vi "Initialize Waveforms V4.vi"(0 "Image Acquisition Parameters":T2={"Scan Type"=enum."Sample Scanning", "Scan Mode"=enum."XY", "Fast Axis Frequency (Hz)"=100.0, "Image Format"=128, "Line Accumulations"=1, "Frames Per Capture"=1, "Frames Accumulations"=1, "Image Dimension (um)"=[], "Number of Z Steps"=1, "Z Steps Size (um)"=1.0, "Pixel Size (nm)"=[], "Customized Image Format"=[]} {"Z Steps Size (um)" min=0.0; "Number of Z Steps" min=1; "Frames Accumulations" min=1; "Frames Per Capture" min=1; "Line Accumulations" min=1; "Image Format" items=["64 x 64"=64, "128 x 128"=128, "256 x 256"=256, "512 x 512"=512, "1024 x 1024"=1024, "2048 x 2048"=2048, "Customized..."=0]}) -> (4 "Waveform Data to FPGA":T1)   [LabVIEW 2014]
uses:
  Type Defs/Image Acquisition Parameters.ctl
  Waveform Data.ctl
panel:
  in  "Slow Axis 2 Delay (Galvo - Not YZ)":i32=2
  in  "Number Data of Points":i32=5000
  # "Length"
  # "Height"
  # "XY"
  # "Z"
  # "Length"
  # "Height"
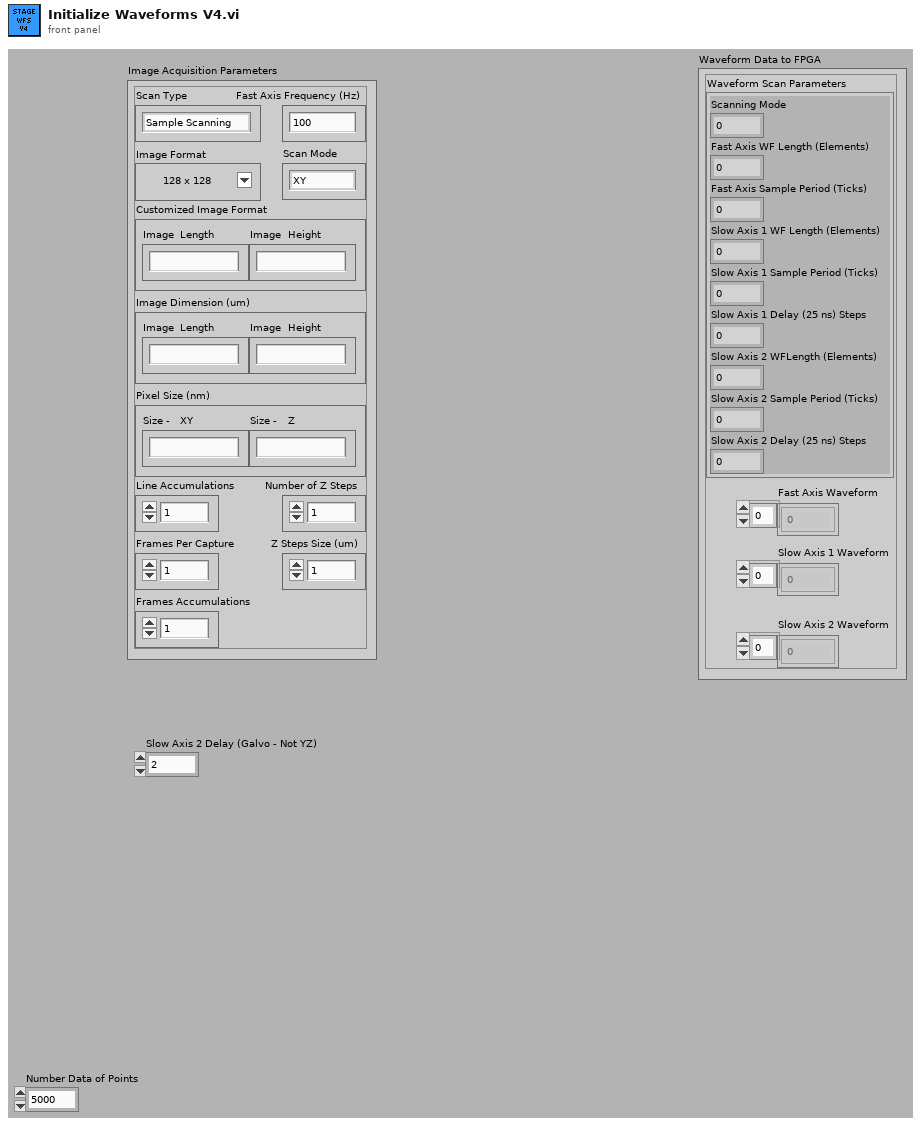
[diagram p1: front panel]
types:
  T1 = typedef "Waveform Data.ctl" = cluster{"Waveform Scan Parameters":cluster{"Scanning Mode":u8, "Fast Axis WF Length (Elements)":i32, "Fast Axis Sample Period (Ticks)":u32, "Slow Axis 1 WF Length (Elements)":i32, "Slow Axis 1 Sample Period (Ticks)":u32, "Slow Axis 1 Delay (25 ns) Steps":i32, "Slow Axis 2 WFLength (Elements)":i32, "Slow Axis 2 Sample Period (Ticks)":u32, "Slow Axis 2 Delay (25 ns) Steps":i32}, "Fast Axis Waveform":dbl[], "Slow Axis 1 Waveform":dbl[], "Slow Axis 2 Waveform":dbl[]}
  T2 = typedef "Image Acquisition Parameters.ctl" = cluster{"Scan Type":enum16{"Sample Scanning", "Beam Scanning"}, "Scan Mode":enum16{"XY", "XZ", "YZ", "XYZ"}, "Fast Axis Frequency (Hz)":dbl, "Image Format":u16, "Line Accumulations":u16, "Frames Per Capture":u16, "Frames Accumulations":u16, "Image Dimension (um)":dbl[], "Number of Z Steps":u8, "Z Steps Size (um)":dbl, "Pixel Size (nm)":dbl[], "Customized Image Format":dbl[]}
  T3 = cluster{"Scanning Mode":u8, "Fast Axis WF Length (Elements)":i32, "Fast Axis Sample Period (Ticks)":u32, "Slow Axis 1 WF Length (Elements)":i32, "Slow Axis 1 Sample Period (Ticks)":u32, "Slow Axis 1 Delay (25 ns) Steps":i32, "Slow Axis 2 WFLength (Elements)":i32, "Slow Axis 2 Sample Period (Ticks)":u32, "Slow Axis 2 Delay (25 ns) Steps":i32}
  T4 = typedef "Scan Parameters.ctl" = cluster{"Fast_Ax_Amp_V":dbl, "Fast_Ax_Off_V":dbl, "Slow_Ax_Amp_V":dbl, "Slow_Ax_Off_V ":dbl, "Slow_Ax_Max_V_VperS":dbl, "Slow_Ax1_Del25ns":i32, "Slow_Ax2_Del25ns":i32, "Stage_X_Off_V":dbl, "Stage_Y_Off_V":dbl, "Stage_Z_Off_V":dbl, "Galvo1_Off_V":dbl, "Galvo2_Off_V":dbl, "Last_Scan_Mode":enum16{"XY", "XZ", "YZ", "XYZ"}, "Current_Scan_Mode":enum16{"XY", "XZ", "YZ", "XYZ"}, "Fly_Back_Lines":u16, "Linear_Ramp_End":u32, "Z_Step_I16":i16, "Z_Start_I16":i16, "Laser_States _U32":u32, "590_Voltage_I16":i16, "775_AOM_Volt_I16":i16, "Blanking OFF":bool, "Unused_Axis_I16":i16}
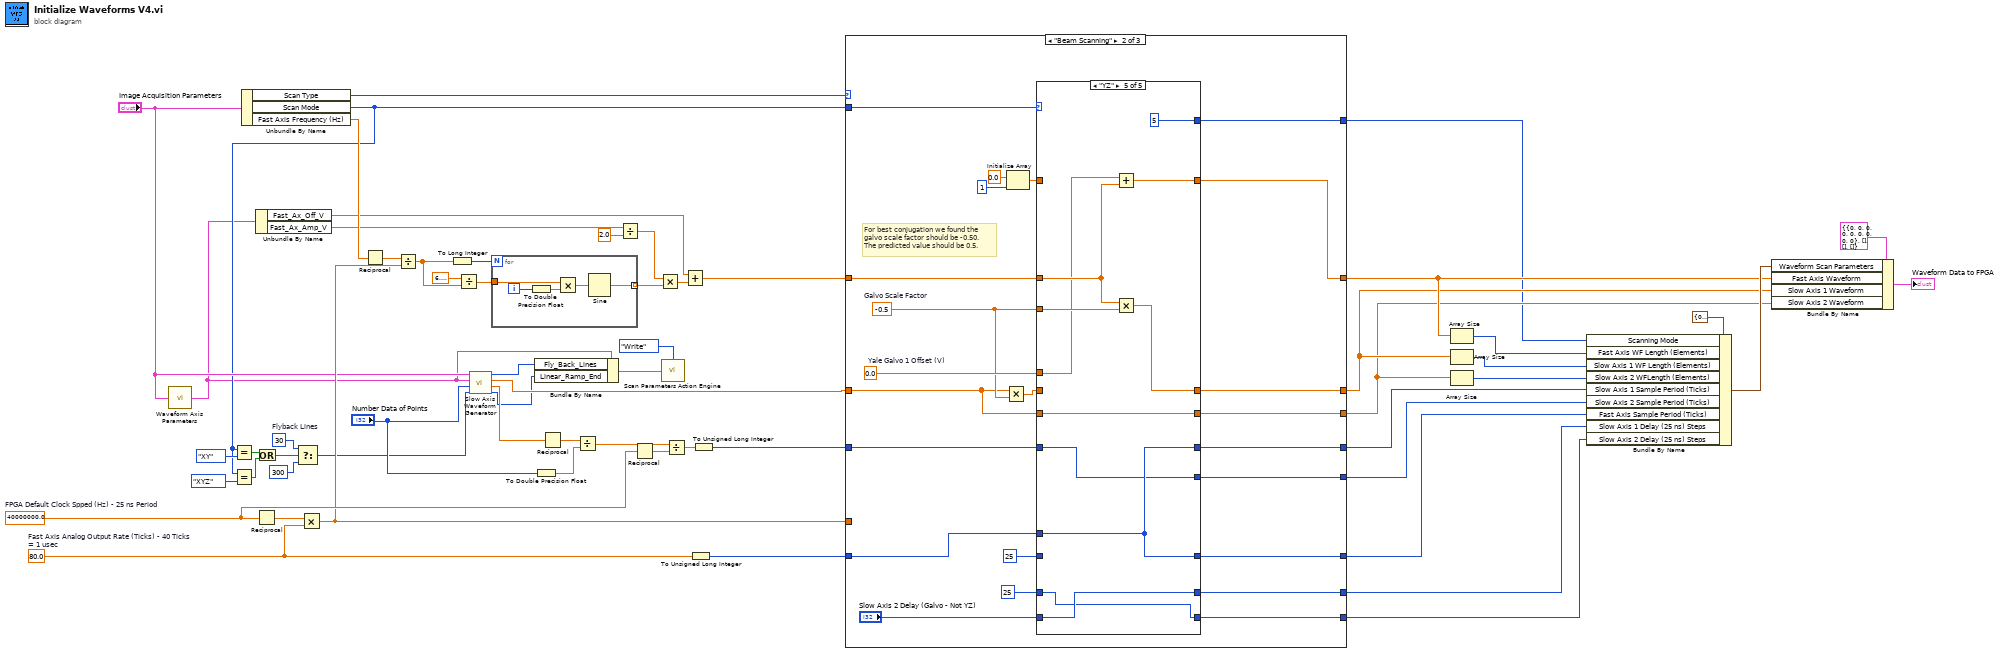
[diagram p0: block diagram]
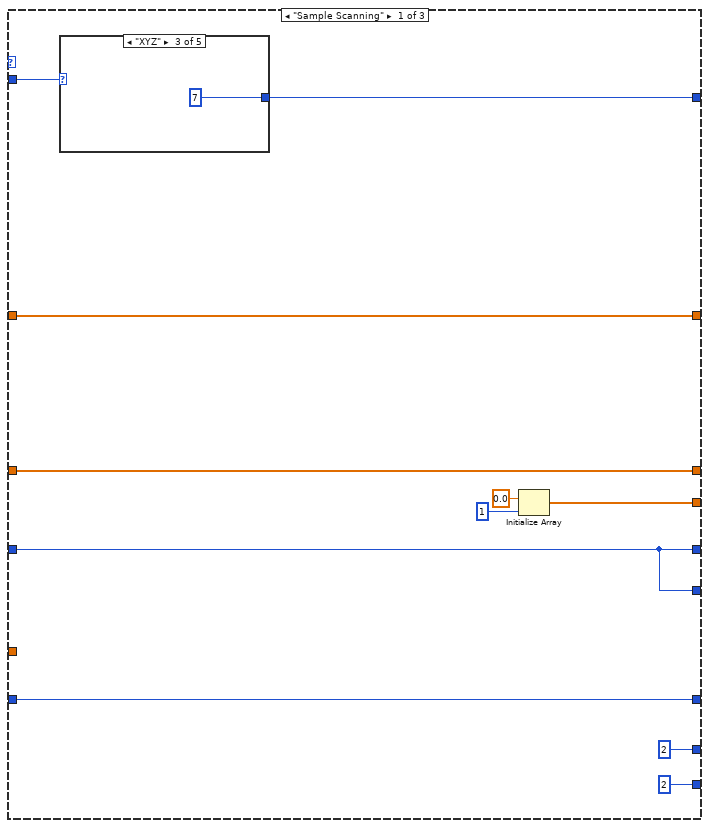
[diagram p2: hidden frame]
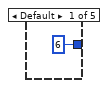
[diagram p3: hidden frame]
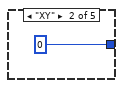
[diagram p4: hidden frame]
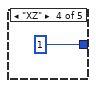
[diagram p5: hidden frame]
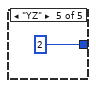
[diagram p6: hidden frame]
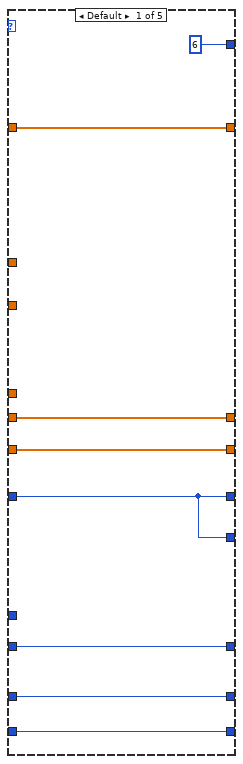
[diagram p7: hidden frame]
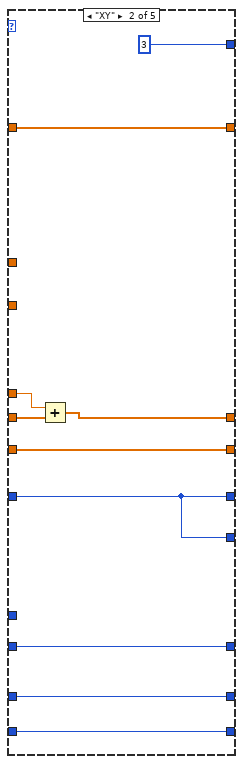
[diagram p8: hidden frame]
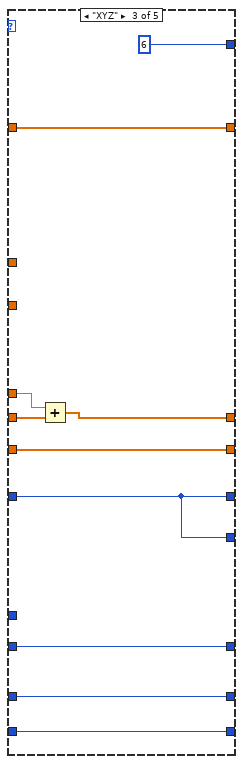
[diagram p9: hidden frame]
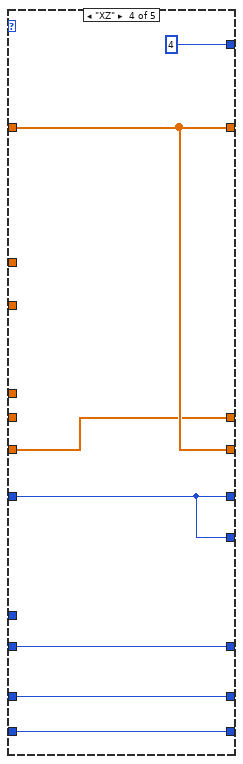
[diagram p10: hidden frame]
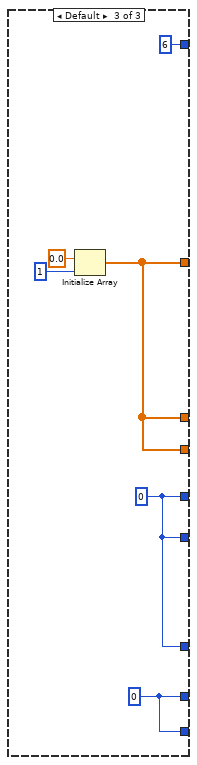
[diagram p11: hidden frame]
diagram:
  w10 = u16 30  # Flyback Lines
  w36 = 80.0  # Fast Axis Analog Output Rate (Ticks) - 40 Ticks = 1 usec
  w46 = 40000000.0  # FPGA Default Clock Spped (Hz) - 25 ns Period
  n1 = call "Waveform Axis Parameters.vi"("Image Acquisition Parameters"="Image Acquisition Parameters") -> ("Scan Parameters"=w1:T4)  [unwired: 14 in]
  n2 = Unbundle By Name("Image Acquisition Parameters") -> ("Scan Type"=w51:enum16{"Sample Scanning", "Beam Scanning"}, "Scan Mode"=w2:enum16{"XY", "XZ", "YZ", "XYZ"}, "Fast Axis Frequency (Hz)"=w21:dbl)
  n3 = Equal?(x=w2, y=enum16{"XY", "XZ", "YZ", "XYZ"}."XY") -> (x = y?=w6:bool)
  n4 = Equal?(x=w2, y=enum16{"XY", "XZ", "YZ", "XYZ"}."XYZ") -> (x = y?=w5:bool)
  n5 = Unbundle By Name(w1) -> ("Fast_Ax_Off_V"=w18:dbl, "Fast_Ax_Amp_V"=w19:dbl)
  n6 = Reciprocal(x=w46) -> (1/x=w50:dbl)
  n7 = Or(x=w6, y=w5) -> (x .or. y?=w4:bool)
  n8 = Select(t=w10, s=w4, f=u16 300) -> (s? t:f=w3:u16)
  n9 = Multiply(x=w50, y=w36) -> (x*y=w16:dbl)
  n10 = Reciprocal(x=w21) -> (1/x=w26:dbl)
  n11 = Divide(x=w26, y=w16) -> (x/y=w24:dbl)
  n12 = To Long Integer(number=w24) -> (32bit integer=w25:i32)
  n13 = Divide(x=6.283185307179586, y=w24) -> (x/y=w29:dbl)
  n14 = call "Slow Axis Waveform Generator.vi"("Flyback Lines"=w3, "Number Data of Points"="Number Data of Points", "Scan Parameters"=w1, "Image Acquisition Parameters"="Image Acquisition Parameters") -> ("Linear Ramp End"=w12:u32, "Slow Axis Frequency"=w48:dbl, "Slow Axis Waveform"=w49:dbl[], "Flyback Lines"=w15:u16)
  n15 = for {
    N: w25 -> [_]
    tunnel: w29 -> [w64]
    tunnel: [w61] -> w28 mode=indexing
    i -> [w60]
    n16 = To Double Precision Float(number=w60) -> (double precision float=w63:dbl)
    n17 = Multiply(x=w64, y=w63) -> (x*y=w62:dbl)
    n18 = Sine(x=w62) -> (sin(x)=w61:dbl)
  }
  n19 = Bundle By Name(cluster=w1, "Fly_Back_Lines"=w15, "Linear_Ramp_End"=w12) -> (w13:T4)
  n20 = To Double Precision Float(number="Number Data of Points") -> (double precision float=w55:dbl)
  n21 = Reciprocal(x=w48) -> (1/x=w56:dbl)
  n22 = Divide(x=w56, y=w55) -> (x/y=w54:dbl)
  n23 = Divide(x=w19, y=2.0) -> (x/y=w22:dbl)
  n24 = Reciprocal(x=w46) -> (1/x=w53:dbl)
  n25 = Multiply(x=w22, y=w28) -> (x*y=w27:dbl[])
  n26 = call "Scan Parameters Action Engine.vi"("Action"=enum16{"Read", "Write"}."Write", "Scan Parameters IN"=w13) -> ()  [unwired: 13 in, 1 out]
  n27 = Divide(x=w54, y=w53) -> (x/y=w52:dbl)
  n28 = Add(x=w18, y=w27) -> (x+y=w20:dbl[])
  n29 = To Unsigned Long Integer(number=w36) -> (unsigned 32bit integer=w35:u32)
  n30 = To Unsigned Long Integer(number=w52) -> (unsigned 32bit integer=w45:u32)
  n31 = case shown="\"Beam Scanning\"" w51 {
    tunnel: w2 -> [w75 w103 _]
    tunnel: w16 -> [_ _ _]
    tunnel: [w65 w101 w152] -> w43
    tunnel: w49 -> [w74 w81 _]
    tunnel: [w74 w97 w152] -> w42
    tunnel: [w71 w96 w152] -> w41
    tunnel: w45 -> [w68 w87 _]
    tunnel: [w70 w102 u8 6 ("Scanning Mode")] -> w37
    tunnel: w35 -> [w69 w84 _]
    tunnel: [w69 w93 w151] -> w34
    tunnel: [w68 w86 w151] -> w33
    tunnel: [w68 w85 w151] -> w32
    tunnel: [2 ("Slow Axis 2 Delay (25 ns) Steps") w92 w150] -> w31
    tunnel: [2 ("Slow Axis 2 Delay (25 ns) Steps") w90 w150] -> w17
    tunnel: w20 -> [w65 w94 _]
    frame "Sample Scanning" {
      n32 = case shown="\"XYZ\"" w75 {
        tunnel: [u8 6 ("Scanning Mode") u8 0 ("Scanning Mode") u8 7 ("Scanning Mode") u8 1 ("Scanning Mode") u8 2 ("Scanning Mode")] -> w70
        frame Default {
        }
        frame "XY" {
        }
        frame "XYZ" {
        }
        frame "XZ" {
        }
        frame "YZ" {
        }
      }
      n33 = Initialize Array(0.0 ("element"), 1 ("dimension size")) -> (w71:dbl[])
    }
    frame "Beam Scanning" {
      w82 = -0.5  # Galvo Scale Factor
      w95 = 0.0  # Yale Galvo 1 Offset (V)
      # "For best conjugation we found the\ngalvo scale factor should be -0.50.\nThe predicted value should be 0.5."
      n34 = Multiply(x=w81, y=w82) -> (x*y=w83:dbl[])
      n35 = Initialize Array(0.0 ("element"), 1 ("dimension size")) -> (w98:dbl[])
      n36 = case shown="\"YZ\"" w103 {
        tunnel: [u8 6 ("Scanning Mode") u8 3 ("Scanning Mode") u8 6 ("Scanning Mode") u8 4 ("Scanning Mode") u8 5 ("Scanning Mode")] -> w102
        tunnel: [w110 w120 w130 w137 w144] -> w101
        tunnel: w98 -> [w110 w120 w130 w137 _]
        tunnel: [w109 w117 w127 w132 w148] -> w97
        tunnel: w83 -> [w109 w118 w128 _ _]
        tunnel: w81 -> [w108 w119 w129 w132 w139]
        tunnel: [w108 w119 w129 w137 w139] -> w96
        tunnel: w95 -> [_ w116 w126 _ w145]
        tunnel: w94 -> [_ _ _ _ w146]
        tunnel: w82 -> [_ _ _ _ w147]
        tunnel: [w107 w115 w125 w135 w142] -> w93
        tunnel: u32 25 -> [w107 w115 w125 w135 _]
        tunnel: [w105 w114 w124 w133 w140] -> w92
        tunnel: "Slow Axis 2 Delay (Galvo - Not YZ)" -> [w105 w114 w124 w133 w143]
        tunnel: [w106 w113 w123 w134 w143] -> w90
        tunnel: 25 ("Slow Axis 1 Delay (25 ns) Steps") -> [w106 w113 w123 w134 w140]
        tunnel: [w104 w112 w122 w136 w142] -> w86
        tunnel: w87 -> [w104 w112 w122 w136 w141]
        tunnel: [w104 w112 w122 w136 w141] -> w85
        tunnel: w84 -> [_ _ _ _ w142]
        frame Default {
        }
        frame "XY" {
          n37 = Add(x=w116, y=w118) -> (x+y=w117:dbl[])
        }
        frame "XYZ" {
          n38 = Add(x=w126, y=w128) -> (x+y=w127:dbl[])
        }
        frame "XZ" {
        }
        frame "YZ" {
          n39 = Add(x=w145, y=w146) -> (x+y=w144:dbl[])
          n40 = Multiply(x=w146, y=w147) -> (x*y=w148:dbl[])
        }
      }
    }
    frame Default {
      w150 = 0 ("Slow Axis 2 Delay (25 ns) Steps")
      w151 = u32 0
      n41 = Initialize Array(0.0 ("element"), 1 ("dimension size")) -> (w152:dbl[])
    }
  }
  n42 = Array Size(array=w43) -> (size(s)=w40:i32)
  n43 = Array Size(array=w42) -> (size(s)=w39:i32)
  n44 = Array Size(array=w41) -> (size(s)=w38:i32)
  n45 = Bundle By Name(cluster=T3 {"Scanning Mode"=0, "Fast Axis WF Length (Elements)"=0, "Fast Axis Sample Period (Ticks)"=0, "Slow Axis 1 WF Length (Elements)"=0, "Slow Axis 1 Sample Period (Ticks)"=0, "Slow Axis 1 Delay (25 ns) Steps"=0, "Slow Axis 2 WFLength (Elements)"=0, "Slow Axis 2 Sample Period (Ticks)"=0, "Slow Axis 2 Delay (25 ns) Steps"=0} ("Waveform Scan Parameters"), "Scanning Mode"=w37, "Fast Axis WF Length (Elements)"=w40, "Slow Axis 1 WF Length (Elements)"=w39, "Slow Axis 2 WFLength (Elements)"=w38, "Slow Axis 1 Sample Period (Ticks)"=w33, "Slow Axis 2 Sample Period (Ticks)"=w32, "Fast Axis Sample Period (Ticks)"=w34, "Slow Axis 1 Delay (25 ns) Steps"=w17, "Slow Axis 2 Delay (25 ns) Steps"=w31) -> (w44:T3)
  n46 = Bundle By Name(cluster=T1 {"Waveform Scan Parameters"={"Scanning Mode"=0, "Fast Axis WF Length (Elements)"=0, "Fast Axis Sample Period (Ticks)"=0, "Slow Axis 1 WF Length (Elements)"=0, "Slow Axis 1 Sample Period (Ticks)"=0, "Slow Axis 1 Delay (25 ns) Steps"=0, "Slow Axis 2 WFLength (Elements)"=0, "Slow Axis 2 Sample Period (Ticks)"=0, "Slow Axis 2 Delay (25 ns) Steps"=0}, "Fast Axis Waveform"=[], "Slow Axis 1 Waveform"=[], "Slow Axis 2 Waveform"=[]} ("Waveform Data"), "Waveform Scan Parameters"=w44, "Fast Axis Waveform"=w43, "Slow Axis 1 Waveform"=w42, "Slow Axis 2 Waveform"=w41) -> (→"Waveform Data to FPGA":T1)
